vi "Destruct.vi"(8 "error in (no error)":errorcluster, 11 "Tag in":refnum<class "Tag.lvclass">) -> (0 "error out":errorcluster)   [LabVIEW 2020, in "Tag Engine Core.lvlib" / "Tag.lvclass"]
doc: "_SubVI_"
uses:
  Tag.lvclass
  Tag.lvclass/Tag.ctl
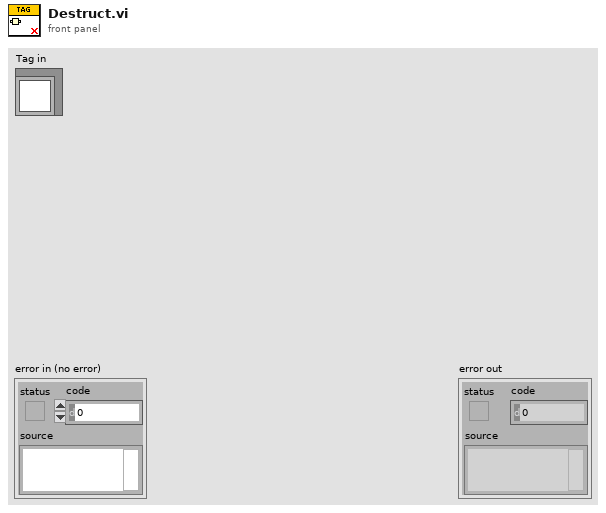
[diagram p1: front panel]
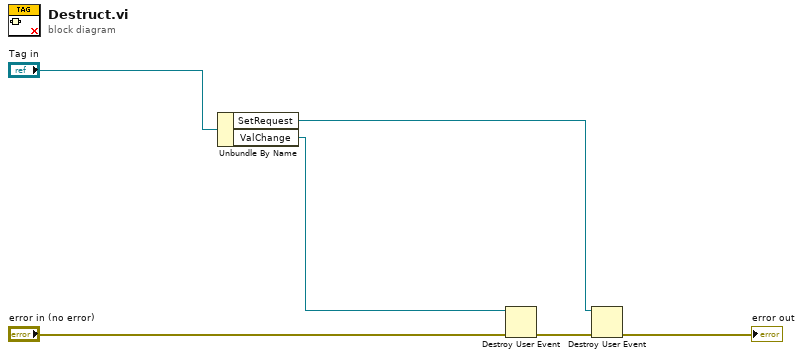
[diagram p0: block diagram]
diagram:
  n1 = Unbundle By Name("Tag in") -> ("SetRequest"=w2:refnum<user-event>, "ValChange"=w4:refnum<user-event>)
  n2 = Destroy User Event(user event=w4, error in="error in (no error)") -> (error out=w3:errorcluster)
  n3 = Destroy User Event(user event=w2, error in=w3) -> (error out=→"error out":errorcluster)
